vi "Measurement Logic.vi"() -> ()   [LabVIEW 2021, in "SourceMeasureDCVoltage.lvlib"]
uses:
  SourceMeasureDCVoltage.lvlib
  Measurement Results.ctl
  Measurement Configuration.ctl
  <vilib>/Plug-In SDKs/Measurements/Measure Call Context/Measure Call Context.lvclass
  FAL/Instruments/Abstract_Instrument/TypeDef/Initialize_Info.ctl
  <vilib>/Plug-In SDKs/Clients/Session Management V1/Session Reservation/Initialize and Close Session Behavior.ctl
  FAL/Instruments/Abstract_Instrument/Utility/Initialize N Pins.vi
  FAL/Functions/Source_Voltage/Utility/Get 1 Object.vi
  FAL/Functions/Measure_Voltage/Utility/Get 1 Object.vi
  FAL/Functions/Source_Voltage/Source_Voltage.lvclass
  FAL/Functions/Measure_Voltage/Measure_Voltage.lvclass
  FAL/Instruments/Abstract_Instrument/Abstract_Instrument.lvclass
  <vilib>/Plug-In SDKs/Clients/Session Management V1/Session Reservation/Session Reservation.lvclass
panel:
  out "measure call context out":refnum<class "Measure Call Context.lvclass">
  in  "measure call context in":refnum<class "Measure Call Context.lvclass">
  in  "measurement configuration":T1={"source_pin"="", "Voltage Level"=0.0, "Voltage Level Range"=0.0, "Current Limit"=0.0, "Current Limit Range"=0.0, "Source Delay (Sec)"=0.0, "measure_pin"="", "Resolution in Digits"=enum."5 1/2"}
  out "measurement results":T2 {"Measurement" format="%.6p"}
  out "error out":errorcluster
  in  "error in":errorcluster
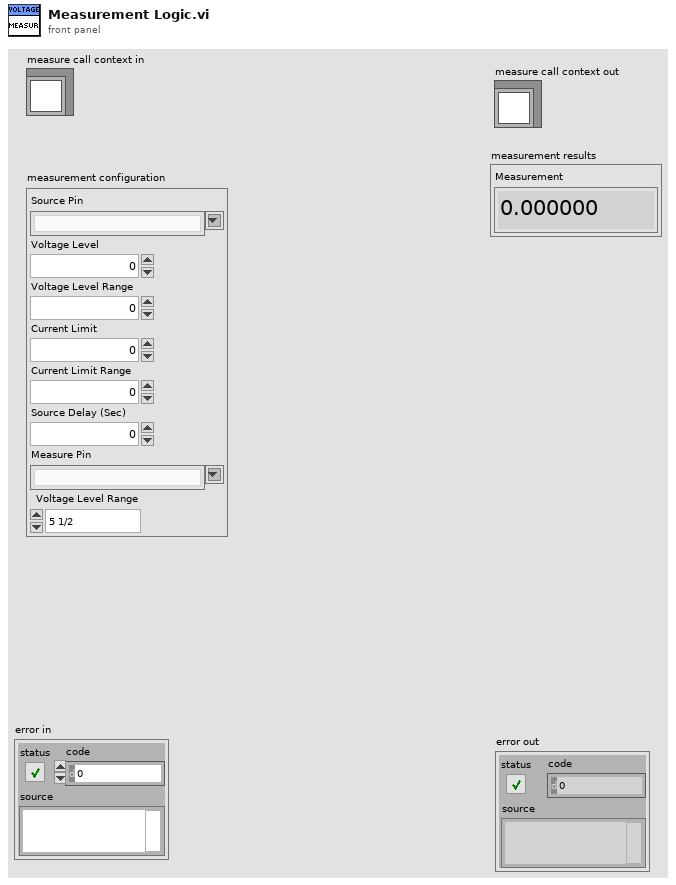
[diagram p1: front panel]
types:
  T1 = typedef "SourceMeasureDCVoltage.lvlib/Measurement Configuration.ctl" = cluster{"source_pin":string, "Voltage Level":dbl, "Voltage Level Range":dbl, "Current Limit":dbl, "Current Limit Range":dbl, "Source Delay (Sec)":dbl, "measure_pin":string, "Resolution in Digits":enum32{"3 1/2", "4 1/2", "5 1/2", "6 1/2", "7 1/2"}}
  T2 = typedef "SourceMeasureDCVoltage.lvlib/Measurement Results.ctl" = cluster{"Measurement":dbl}
  T3 = typedef "NI Session Management V1 Client.lvlib/Session Reservation.lvclass/Initialize and Close Session Behavior.ctl" = enum16{"Auto", "Initialize and Close", "Attach and Detach", "Initialize and Detach", "Attach and Close"}
  T4 = typedef "Abstract_Instrument.lvclass/Initialize_Info.ctl" = cluster{"initialize and close session behavior":T3, "reset":bool, "optional string":string}
  T5 = enum32{"3 1/2", "4 1/2", "5 1/2", "6 1/2", "7 1/2"}
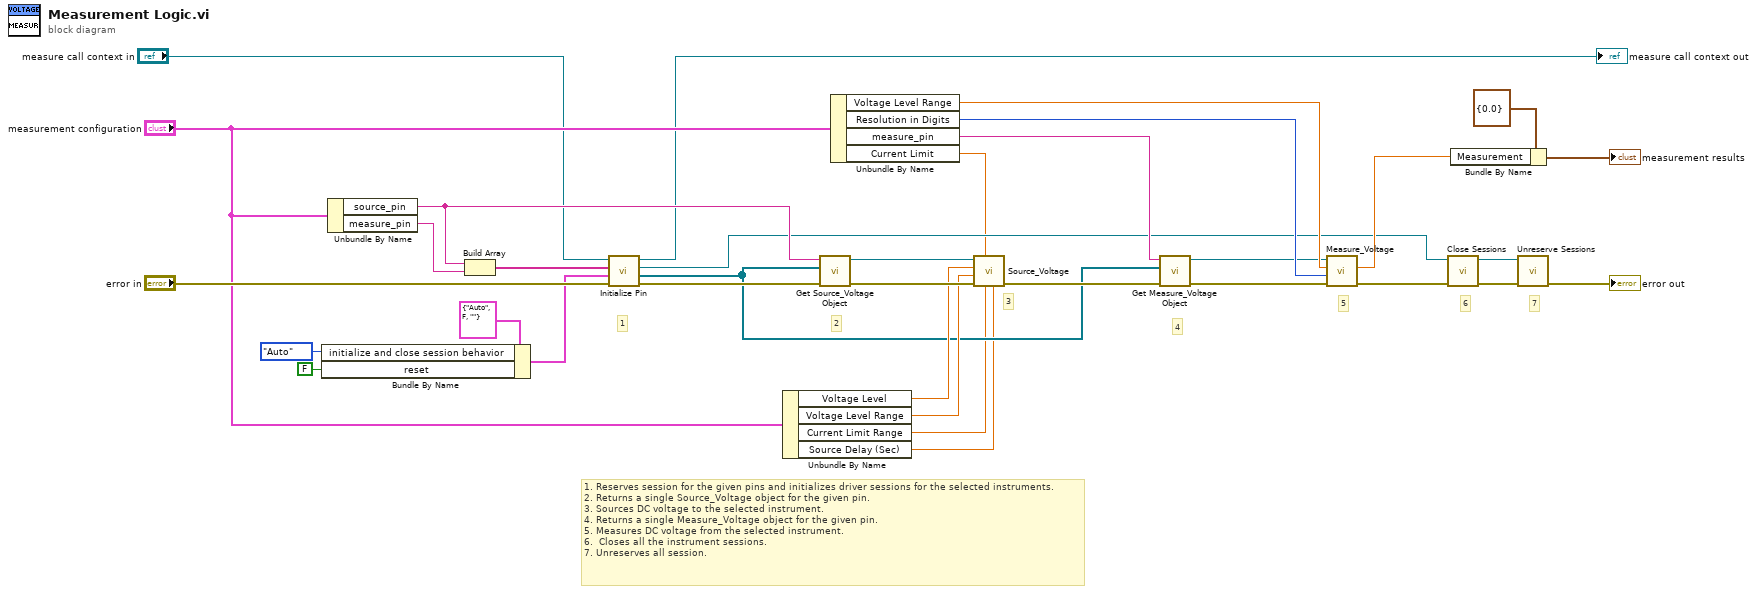
[diagram p0: block diagram]
diagram:
  # "1. Reserves session for the given pins and initializes driver sessions for the selected instruments.\n2. Returns a single Source_Voltage object for the given pin.\n3. Sources DC voltage to the selected instrument.\n4. Returns a single Measure_Voltage object for the given pin.\n5. Measures DC voltage from the selected instrument.\n6.  Closes all the instrument sessions.\n7. Unreserves all session."
  # "7"
  # "6"
  # "5"
  # "4"
  # "3"
  # "2"
  # "1"
  n1 = Bundle By Name(cluster=T4 {"initialize and close session behavior"=enum."Auto", "reset"=FALSE, "optional string"=""} ("Initialize_Info"), "initialize and close session behavior"=Initialize_and_Close_Session_Behavior."Auto", "reset"=FALSE) -> (w8:T4)
  n2 = Unbundle By Name("measurement configuration") -> ("source_pin"=w20:string, "measure_pin"=w23:string)
  n3 = Build Array(w20, w23) -> (w21:string[])
  n4 = call-poly "Initialize Pin.vi"("error in"="error in", "Initialize_Info"=w8, "pin or relay names"=w21, "measure call context in"="measure call context in") -> ("error out"=w22:errorcluster, "instrument object"=w17:refnum<class "Abstract_Instrument.lvclass">[], "session reservation out"=w15:refnum<class "Session Reservation.lvclass">, "measure call context out"=→"measure call context out":refnum<class "Measure Call Context.lvclass">)  [unwired: 4 in]
  n5 = Unbundle By Name("measurement configuration") -> ("Voltage Level"=w25:dbl, "Voltage Level Range"=w24:dbl, "Current Limit Range"=w5:dbl, "Source Delay (Sec)"=w4:dbl)
  n6 = call-poly "Get Source_Voltage Object.vi"("error in"=w22, "instrument object"=w17, "pin_name"=w20) -> ("error out"=w27:errorcluster, "function object"=w19:refnum<class "Source_Voltage.lvclass">)  [unwired: 7 in]
  n7 = Unbundle By Name("measurement configuration") -> ("Voltage Level Range"=w31:dbl, "Resolution in Digits"=w30:T5, "measure_pin"=w18:string, "Current Limit"=w6:dbl)
  n8 = call-dynamic "Source_Voltage.vi"("Source Delay (Sec)"=w4, "Current Limit Range"=w5, "Current Limit"=w6, "error in (no error)"=w27, "Voltage Level Range"=w24, "Voltage Level"=w25, "Source_Voltage in"=w19) -> ("error out"=w26:errorcluster)  [unwired: 3 in, 1 out]
  n9 = call-poly "Get Measure_Voltage Object.vi"("error in"=w26, "instrument object"=w17, "pin_name"=w18) -> ("error out"=w28:errorcluster, "function object"=w16:refnum<class "Measure_Voltage.lvclass">)  [unwired: 7 in]
  n10 = call-dynamic "Measure_Voltage.vi"("error in (no error)"=w28, "Resolution in Digits"=w30, "Range"=w31, "Measure_Voltage in"=w16) -> ("error out"=w32:errorcluster, "DC_Voltage"=w29:dbl)  [unwired: 4 in, 2 out]
  n11 = call <vilib>:"Close Sessions.vi"("error in"=w32, "session reservation in"=w15) -> ("error out"=w34:errorcluster, "session reservation out"=w33:refnum<class "Session Reservation.lvclass">)  [unwired: 8 in]
  n12 = Bundle By Name(cluster=T2 {"Measurement"=0.0} ("measurement results"), "Measurement"=w29) -> (→"measurement results":T2)
  n13 = call <vilib>:"Unreserve Sessions.vi"("error in"=w34, "session reservation in"=w33) -> ("error out"=→"error out":errorcluster)  [unwired: 9 in]
